vi "Read Temperature.vi"(0 "Session Handle":T2, 5 "Pelt Temp Sensors":T1=49 items=["PTS1"=49, "PTS2"=50, "PTS3"=51, "PTS4"=52, "PTS5"=53, "PTS6"=54], 11 "error in (no error)":errorcluster) -> (4 "Session Handle Out":T2, 6 "Temperature":dbl, 15 "error out":errorcluster)   [LabVIEW 2015, in "Peltier.lvclass"]
uses:
  Peltier.lvclass
  Typedefs/Session Handle.ctl
  Typedefs/Peltier Temperature Sensors.ctl
  Gas/Gas.lvclass
panel:
  out "Success?":bool
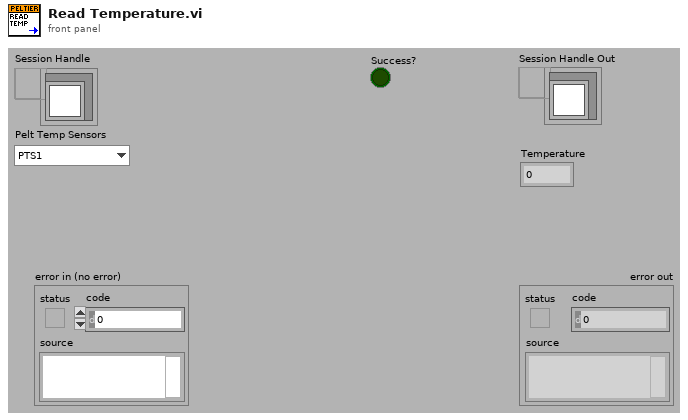
[diagram p1: front panel]
types:
  T1 = typedef "Peltier.lvclass/Peltier Temperature Sensors.ctl" = u16
  T2 = typedef "Peltier.lvclass/Session Handle.ctl" = refnum<data-value>
  T3 = typedef "XNET Frame CAN.ctl" = cluster{"timestamp":timestamp, "payload":u8[], "identifier":u32, "type":T4, "extended?":bool, "echo?":bool}
  T4 = typedef "XNET Frame Type CAN.ctl" = u8
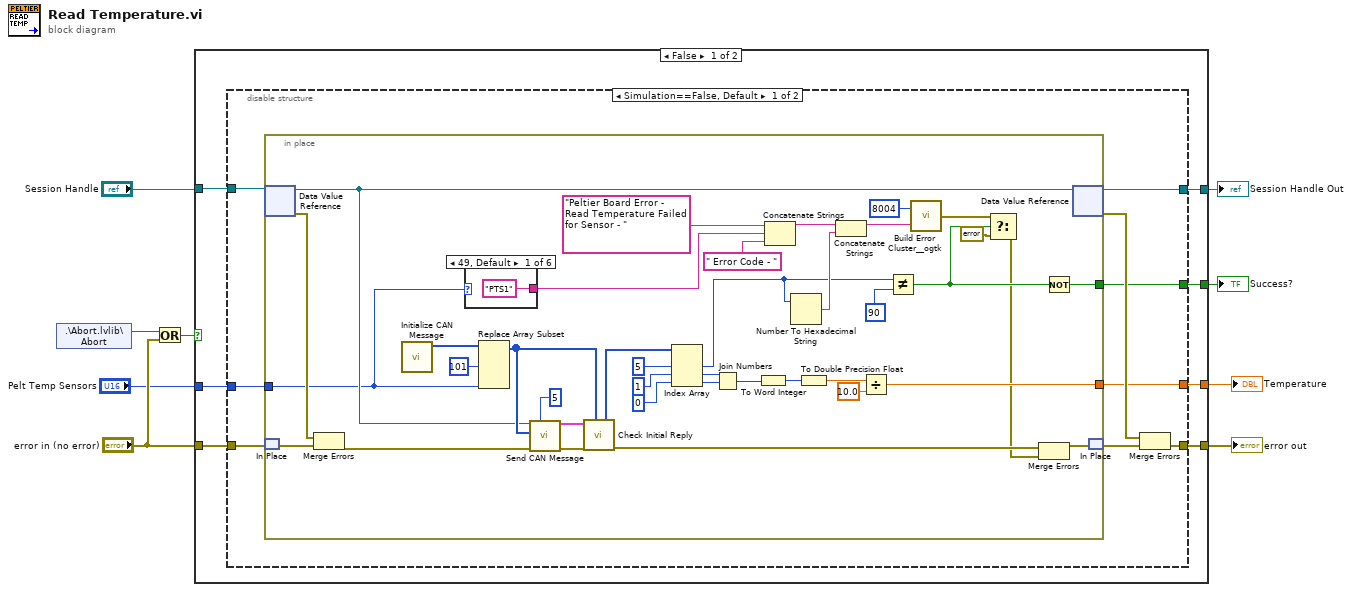
[diagram p0: block diagram]
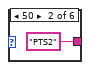
[diagram p2: hidden frame]
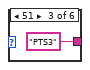
[diagram p3: hidden frame]
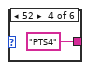
[diagram p4: hidden frame]
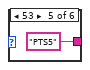
[diagram p5: hidden frame]
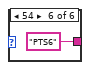
[diagram p6: hidden frame]
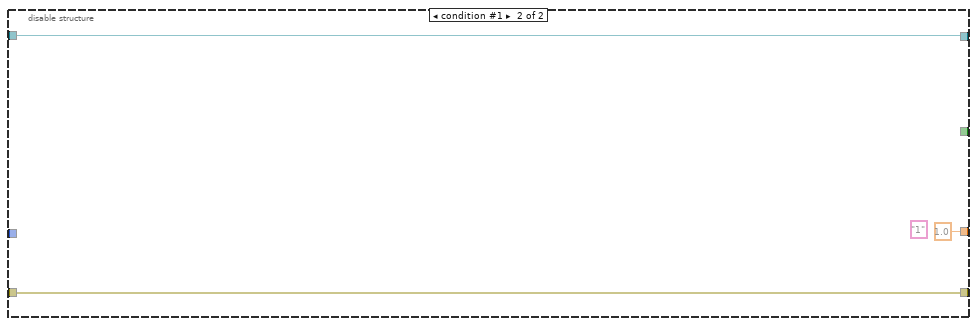
[diagram p7: hidden frame]
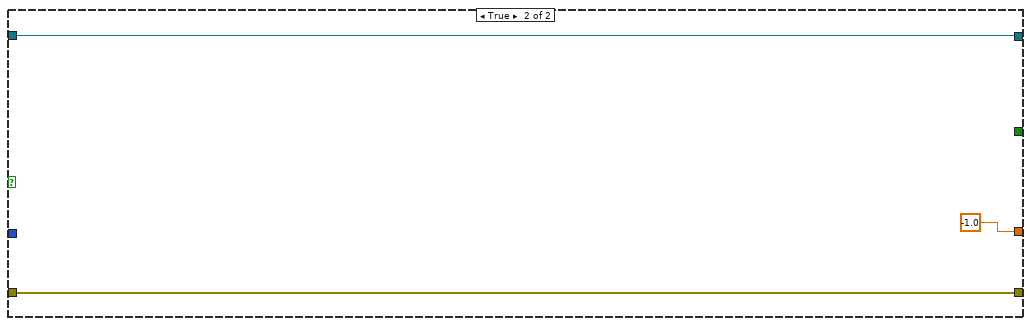
[diagram p8: hidden frame]
diagram:
  n1 = shared-variable ".\\Abort.lvlib\\Abort"() -> (w8:bool)  [unwired: 1 in, 1 out]
  n2 = Or(x=w8, y="error in (no error)") -> (x .or. y?=w6:bool)
  n3 = case shown="False" w6 {
    tunnel: [w16 w75] -> w2
    tunnel: [w15 w74] -> w9
    tunnel: "Session Handle" -> [w14 w75]
    tunnel: "error in (no error)" -> [w13 w74]
    tunnel: [w12 -1.0] -> w5
    tunnel: [w11 _] -> w4
    tunnel: "Pelt Temp Sensors" -> [w10 _]
    frame False {
      n4 = disable-structure shown="Simulation==False, Default" {
        disable-tunnel: [w25 w72] -> w16
        disable-tunnel: [w22 w71] -> w15
        disable-tunnel: w14 -> [w21 w72]
        disable-tunnel: w13 -> [w20 w71]
        disable-tunnel: [w19 1.0] -> w12
        disable-tunnel: [w18 _] -> w11
        disable-tunnel: w10 -> [w17 _]
        frame condition #0 (active) {
          n5 = in-place {
            in-place-border: [w37] -> w19
            in-place-border: [w46] -> w18
            in-place-border: w17 -> [w30]
            n6 = in-place-dvr #1(w21) -> (w54:refnum<class "Peltier.lvclass">, w59:errorcluster)
            n7 = in-place-match #2(w20) -> (w58:errorcluster)
            n8 = Merge Errors(w59, w58) -> (w53:errorcluster)
            n9 = call "Initialize CAN Message.vi"() -> ("Initial Payload"=w61:u8[])  [unwired: 11 in]
            n10 = case shown="49, Default" w30 {
              tunnel: ["PTS1" "PTS2" "PTS3" "PTS4" "PTS5" "PTS6"] -> w28
              frame 49, Default {
              }
              frame 50 {
              }
              frame 51 {
              }
              frame 52 {
              }
              frame 53 {
              }
              frame 54 {
              }
            }
            n11 = Replace Array Subset(array=w61, new element #1=u8 101 ("new element/subarray"), new element #2=w30) -> (w57:u8[])  [unwired: 2 in]
            n12 = call "Send CAN Message.vi"("Number of Retries"=5, "error in (no error)"=w53, "payload"=w57, "Peltier In"=w54) -> ("error out"=w33:errorcluster, "Reply"=w55:T3[])  [unwired: 5 in, 1 out]
            n13 = call "Check Initial Reply.vi"("Write Message"=w57, "error in (no error)"=w33, "Reply"=w55) -> ("error out"=w32:errorcluster, "Data Packet"=w60:u8[])  [unwired: 5 in, 2 out]
            n14 = Index Array(array=w60, index #1=5 ("index"), index #2=1 ("index"), index #3=0 ("index")) -> (element #1=w47:u8, element #2=w42:u8, element #3=w41:u8)
            n15 = Join Numbers(hi=w42, lo=w41) -> ((hi.lo)=w40:u16)
            n16 = To Word Integer(number=w40) -> (16bit integer=w43:i16)
            n17 = Concatenate Strings("Peltier Board Error -  Read Temperature Failed for Sensor - " ("string"), w28, " Error Code - ") -> (w26:string)
            n18 = Number To Hexadecimal String(2:w47) -> (0:w51:string)  [unwired: 1 in]
            n19 = To Double Precision Float(number=w43) -> (double precision float=w39:dbl)
            n20 = Concatenate Strings(w26, w51) -> (w50:string)
            n21 = Divide(x=w39, y=10.0) -> (x/y=w37:dbl)
            n22 = Not Equal?(x=w47, y=u8 90 ("new element/subarray")) -> (x != y?=w34:bool)
            n23 = call <userlib>:"Build Error Cluster__ogtk.vi"("String to Prepend to source (\"\")"=w50, "code"=8004) -> ("error out"=w36:errorcluster)
            n24 = Select(t=w36, s=w34, f=errorcluster {"status"=FALSE, "code"=0, "source"=""}) -> (s? t:f=w31:errorcluster)
            n25 = Merge Errors(w32, w31) -> (w62:errorcluster)
            n26 = Not(x=w34) -> (.not. x?=w46:bool)
            n27 = in-place-dvr #1(w54) -> (w25:T2, w23:errorcluster)
            n28 = in-place-match #2(w62) -> (w24:errorcluster)
          }
          n29 = Merge Errors(w23, w24) -> (w22:errorcluster)
        }
        frame condition #1 {
          (unwired) "1"
        }
      }
    }
    frame True {
    }
  }
  "error out" <- w9
  "Temperature" <- w5
  "Success?" <- w4
  "Session Handle Out" <- w2
